vi "Example 5 (Find FPGA Addon).vi"() -> ()   [LabVIEW 2018]
uses:
  <vilib>/addons/VeriStand Custom Device Scripting APIs/FPGA Addon/Scripting API.lvlibp/1abvi3w/vi.lib/NI Veristand/Custom Device API/Custom Device Item Ref.ctl
  <vilib>/addons/VeriStand Custom Device Scripting APIs/FPGA Addon/Scripting API.lvlibp
  <vilib>/addons/VeriStand Custom Device Scripting APIs/FPGA Addon/Scripting API.lvlibp/1abvi3w/vi.lib/NI Veristand/Custom Device API/Custom Device API.lvlib
panel:
  out "FPGA Addons Found ?":bool
  out "FPGA Addon refnums out":T1[](array[typedef]) format="%.0x"
  out "FPGA Addon refnum out":T1=18446744073709551615 format="%.0x"
  out "FPGA Addon Found ?":bool
  out "error out":errorcluster
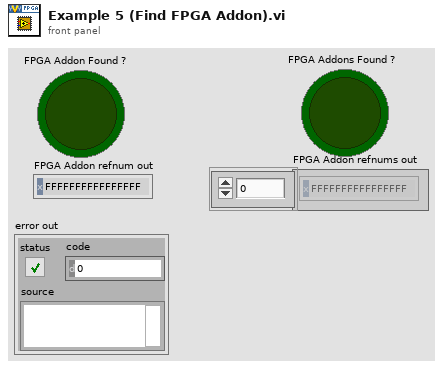
[diagram p1: front panel]
types:
  T1 = typedef "Scripting API.lvlibp/Custom Device API.lvlib/Custom Device Item Ref.ctl" = u64
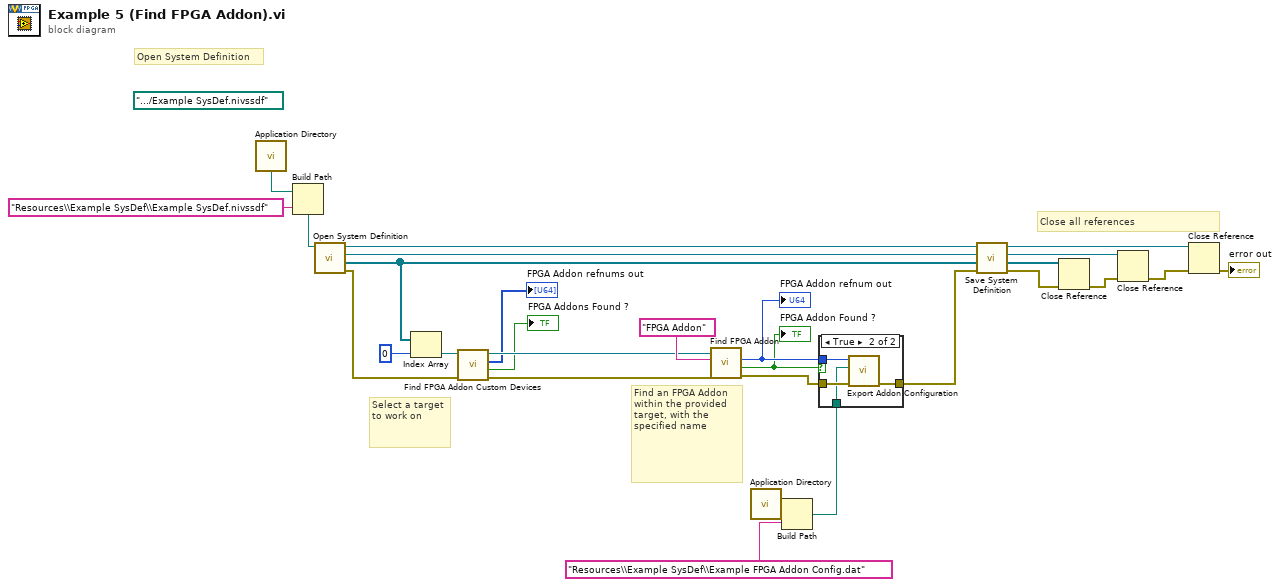
[diagram p0: block diagram]
diagram:
  (unwired) path ".../Example SysDef.nivssdf" ("fpga bitfile path")
  # "Close all references"
  # "Find an FPGA Addon within the provided target, with the specified name"
  # "Select a target to work on"
  # "Open System Definition"
  n1 = call <vilib>:"Application Directory.vi"() -> ("Application Directory"=w21:path)
  n2 = Build Path(base path=w21, name or relative path="Resources\\Example SysDef\\Example SysDef.nivssdf") -> (appended path=w19:path)
  n3 = call "Open System Definition.vi"("System Definition File"=w19) -> ("error out"=w5:errorcluster, "targets refnums"=w24:refnum<k24>[], "root refnum"=w25:refnum<k24>, "system definition refnum"=w17:refnum<k24>)  [unwired: 7 in]
  n4 = Index Array(array=w24, index=0) -> (element=w7:refnum<k24>)
  n5 = call <vilib>:"Find FPGA Addon Custom Devices.vi"("error in (no error)"=w5, "target in"=w7) -> ("error out"=w4:errorcluster, "found ?"=→"FPGA Addons Found ?":bool, "FPGA Addon refnums out"=→"FPGA Addon refnums out":T1[], "target out"=w6:refnum<k24>)  [unwired: 6 in]
  n6 = call <vilib>:"Find FPGA Addon.vi"("error in (no error)"=w4, "FPGA Addon name"="FPGA Addon" ("fpga addon name"), "target in"=w6) -> ("error out"=w12:errorcluster, "found ?"=w1:bool, "FPGA Addon refnum out"=w13:T1)  [unwired: 5 in, 1 out]
  "FPGA Addon Found ?" <- w1
  "FPGA Addon refnum out" <- w13
  n7 = call <vilib>:"Application Directory.vi"() -> ("Application Directory"=w11:path)
  n8 = Build Path(base path=w11, name or relative path="Resources\\Example SysDef\\Example FPGA Addon Config.dat") -> (appended path=w9:path)
  n9 = case shown="True" w1 {
    tunnel: w13 -> [_ w31]
    tunnel: w12 -> [w27 w30]
    tunnel: w9 -> [_ w29]
    tunnel: [w27 w28] -> w8
    frame False {
    }
    frame True {
      n10 = call <vilib>:"Export Addon Configuration.vi"("error in (no error)"=w30, "export file path"=w29, "FPGA Addon refnum in"=w31) -> ("error out"=w28:errorcluster)  [unwired: 7 in, 1 out]
    }
  }
  n11 = call "Save System Definition.vi"("error in (no error)"=w8, ".NET Refnum in"=w17) -> ("error out"=w15:errorcluster, ".NET Refnum out"=w16:refnum<k24>)  [unwired: 8 in]
  n12 = Close Reference(reference=w24, error in (no error)=w15) -> (error out=w23:errorcluster)
  n13 = Close Reference(reference=w25, error in (no error)=w23) -> (error out=w22:errorcluster)
  n14 = Close Reference(reference=w16, error in (no error)=w22) -> (error out=→"error out":errorcluster)
